vi "Parse Parameters File.vi"(8 "error in":errorcluster, 11 "path to XML document":path caption="path to parameters xml") -> (0 "error out":errorcluster, 2 "biu configuration":T1, 3 "path to XML document out":path caption="path to parameters xml")   [LabVIEW 2020, in "AIM MIL-STD 1553 Import.lvlib"]
uses:
  AIM MIL-STD 1553 Import.lvlib
  <resource>/objmgr/DOMUserDefRef.rc
  <vilib>/xml/NI_XML.lvlib
  Constants.vi
  Shared/Address.ctl
  Shared/Message Type.ctl
  Shared/Terminal Endpoint.ctl
  Shared/Parameter Definition.ctl
  Shared/Message Definition.ctl
  Shared/BIU Configuration.ctl
  a98a4505-1d2b-4178-8eef-924facff6c40.vi
  Shared/Minor Frame Definition.ctl
  Shared/Major Frame Definition.ctl
  Shared/Acyclic Frame Definition.ctl
  <vilib>/xml/Load XML File.vi
  <vilib>/xml/Close Reference(Node).vi
  60cc2e63-67cc-4215-8c07-088d80cb97fe.vi
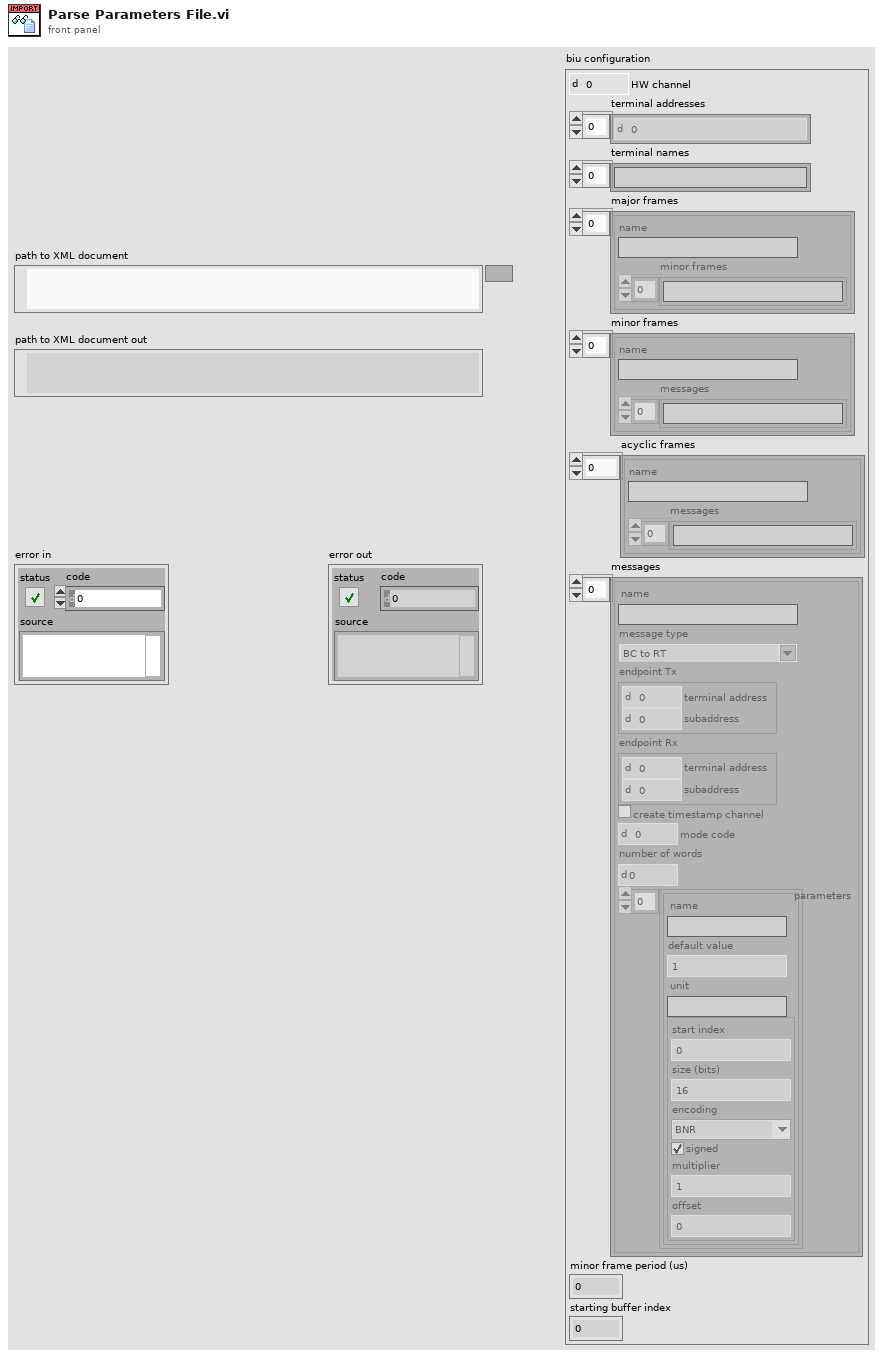
[diagram p1: front panel]
types:
  T1 = typedef "BIU Configuration.ctl" = cluster{"HW channel":u16, "terminal addresses":T2[], "terminal names":string[], "major frames":T3[], "minor frames":T4[], "acyclic frames":T5[], "messages":T6[], "minor frame period (us)":i32, "starting buffer index":u16}
  T2 = typedef "Address.ctl" = u16
  T3 = typedef "Major Frame Definition.ctl" = cluster{"name":string, "minor frames":string[]}
  T4 = typedef "Minor Frame Definition.ctl" = cluster{"name":string, "messages":string[]}
  T5 = typedef "Acyclic Frame Definition.ctl" = cluster{"name":string, "messages":string[]}
  T6 = typedef "Message Definition.ctl" = cluster{"name":string, "message type":T7, "endpoint Tx":T8, "endpoint Rx":T8, "create timestamp channel":bool, "mode code":u16, "number of words":u16, "parameters":cluster{"name":string, "default value":dbl, "unit":string, "parameter definition":T9}[]}
  T7 = typedef "Message Type.ctl" = string
  T8 = typedef "Terminal Endpoint.ctl" = cluster{"terminal address":T2, "subaddress":T2}
  T9 = typedef "Parameter Definition.ctl" = cluster{"start index":i32, "size (bits)":i32, "encoding":enum16{"BNR", "BCD", "Discrete"}, "signed":bool, "multiplier":dbl, "offset":dbl}
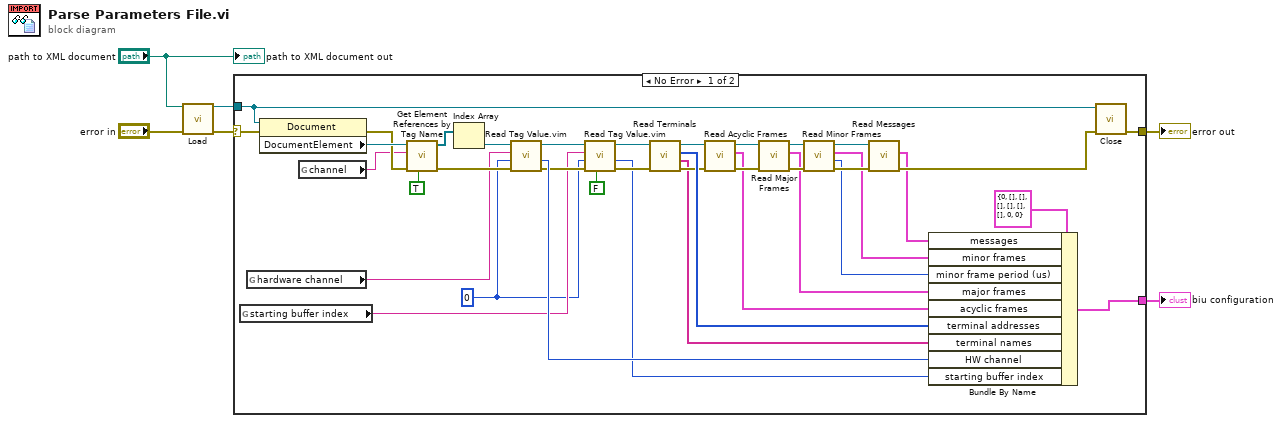
[diagram p0: block diagram]
diagram:
  n1 = call-poly <vilib>:"Load.vi"("path to XML document"="path to XML document", "error in (no error)"="error in") -> ("DOM document out"=w3:refnum<k20>, "error out"=w6:errorcluster)  [unwired: 11 in, 1 out]
  n2 = case shown="No Error" w6 {
    selector: w6 -> [w44 w45]
    tunnel: [w43 w45] -> w4
    tunnel: w3 -> [w42 _]
    tunnel: [w35 _] -> w1
    frame No Error {
      w7 = u16 0
      n3 = global read "Constants.vi" "starting buffer index"() -> (w9:string)
      n4 = global read "Constants.vi" "hardware channel"() -> (w36:string)
      n5 = property class="Document"(reference=w42, error in=w44) -> (error out=w40:errorcluster, "DocumentElement"=w41:refnum<k20>)  [unwired: 1 out]
      n6 = global read "Constants.vi" "channel"() -> (w39:string)
      n7 = call "Get Element References by Tag Name.vi"("required (F)"=TRUE, "error in"=w40, "tag name"=w39, "node in"=w41) -> ("error out"=w38:errorcluster, "array of elements"=w31:refnum<k20>[])  [unwired: 6 in]
      n8 = Index Array(array=w31) -> (element=w32:refnum<k20>)  [unwired: 1 in]
      n9 = call "Read Tag Value.vim"("error in"=w38, "default"=w7, "tag name"=w36, "node in"=w32) -> ("error out"=w14:errorcluster, "value"=w30:u16, "node out"=w13:refnum<k20>)  [unwired: 5 in]
      n10 = call "Read Tag Value.vim"("required (F)"=FALSE, "error in"=w14, "default"=w7, "tag name"=w9, "node in"=w13) -> ("error out"=w11:errorcluster, "value"=w8:u16, "node out"=w12:refnum<k20>)  [unwired: 4 in]
      n11 = call "Read Terminals.vi"("error in"=w11, "channel ref in"=w12) -> ("error out"=w27:errorcluster, "terminal names"=w26:string[], "terminal addresses"=w29:T2[], "channel ref out"=w28:refnum<k20>)  [unwired: 6 in]
      n12 = call "Read Acyclic Frames.vi"("error in"=w27, "channel ref in"=w28) -> ("error out"=w21:errorcluster, "acyclic frames"=w16:T5[], "channel ref out"=w23:refnum<k20>)  [unwired: 7 in]
      n13 = call "Read Major Frames.vi"("error in"=w21, "channel ref in"=w23) -> ("error out"=w20:errorcluster, "major frames"=w17:T3[], "channel ref out"=w22:refnum<k20>)  [unwired: 7 in]
      n14 = call "Read Minor Frames.vi"("error in"=w20, "channel ref in"=w22) -> ("error out"=w24:errorcluster, "minor frame period (us)"=w15:i32, "minor frames"=w18:T4[], "channel ref out"=w25:refnum<k20>)  [unwired: 6 in]
      n15 = call "Read Messages.vi"("error in"=w24, "channel ref in"=w25) -> ("error out"=w34:errorcluster, "messages"=w19:T6[])  [unwired: 7 in, 1 out]
      n16 = Bundle By Name(cluster=T1 {"HW channel"=0, "terminal addresses"=[], "terminal names"=[], "major frames"=[], "minor frames"=[], "acyclic frames"=[], "messages"=[], "minor frame period (us)"=0, "starting buffer index"=0} ("1553 channel"), "messages"=w19, "minor frames"=w18, "minor frame period (us)"=w15, "major frames"=w17, "acyclic frames"=w16, "terminal addresses"=w29, "terminal names"=w26, "HW channel"=w30, "starting buffer index"=w8) -> (w35:T1)
      n17 = call-poly <vilib>:"Close.vi"("error in (no error)"=w34, "node"=w42) -> ("error out"=w43:errorcluster)  [unwired: 7 in]
    }
    frame Error {
    }
  }
  "error out" <- w4
  "biu configuration" <- w1
  "path to XML document out" <- "path to XML document"
